vi "Cam Handler.vi"() -> ()   [LabVIEW 2015]
uses:
  <vilib>/userdefined/High Color/IMAQdx.ctl
  <vilib>/vision/driver/NI_Vision_Acquisition_Software.lvlib
  <resource>/objmgr/imaqdx.rc
  <resource>/objmgr/IMAQImage.rc
panel:
  out "Image Size":cluster{"x":i32, "y":i32}
  in  "stop":bool
  out "error out 2":errorcluster
  out "error out":errorcluster
  out "Image Out":T1(plugin-control)
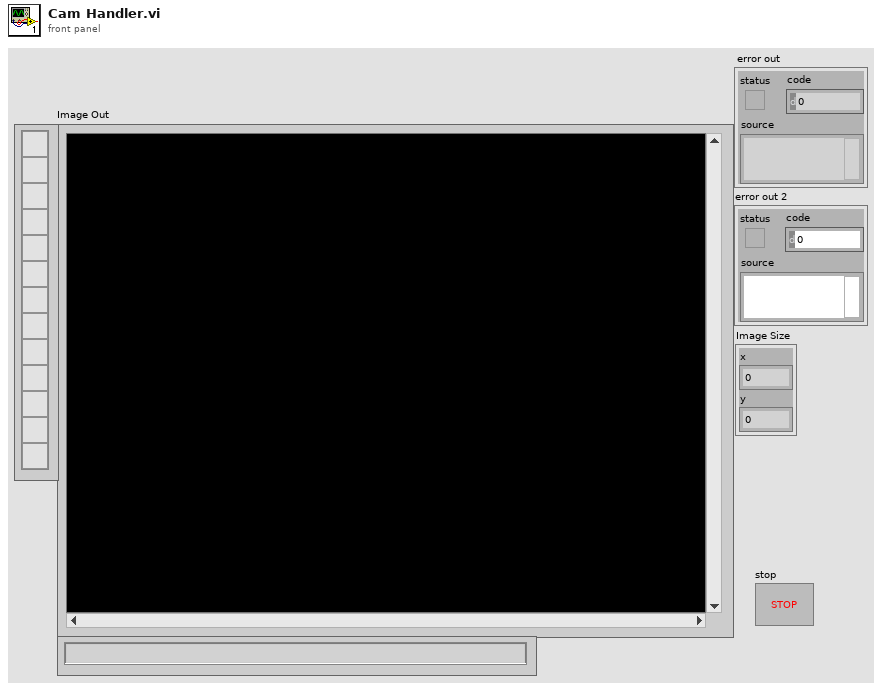
[diagram p1: front panel]
types:
  T1 = typedef "IMAQ Image.ctl" = refnum<image>
  T2 = typedef "IMAQdx.ctl" = refnum<k21>
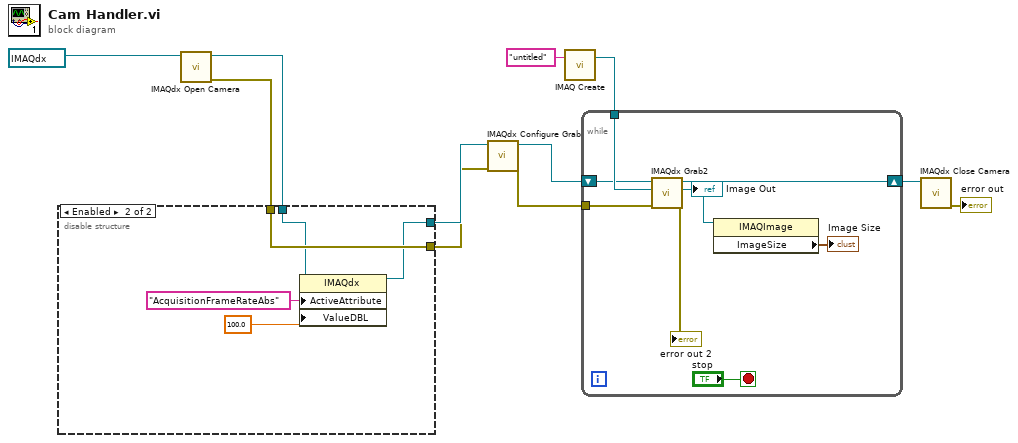
[diagram p0: block diagram]
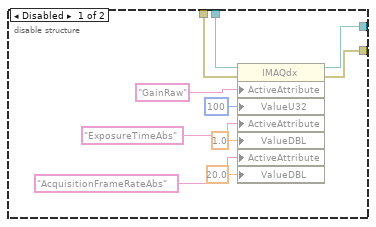
[diagram p2: hidden frame]
diagram:
  n1 = call <vilib>:"IMAQdx Open Camera.vi"("Session In"=T2 "cam1") -> ("error out"=w11:errorcluster, "Session Out"=w10:T2)  [unwired: 9 in]
  n2 = disable-structure shown="Enabled" {
    disable-tunnel: w11 -> [w21 w26]
    disable-tunnel: w10 -> [w20 w25]
    disable-tunnel: [w19 w24] -> w8
    disable-tunnel: [w18 w26] -> w7
    frame Disabled {
      n3 = property class="IMAQdx"(reference=w20, error in=w21, "ActiveAttribute"="GainRaw", "ValueU32"=u32 100, "ActiveAttribute"="ExposureTimeAbs", "ValueDBL"=1.0, "ActiveAttribute"="AcquisitionFrameRateAbs", "ValueDBL"=20.0) -> (reference out=w19:T2, error out=w18:errorcluster)
    }
    frame Enabled {
      n4 = property class="IMAQdx"(reference=w25, "ActiveAttribute"="AcquisitionFrameRateAbs", "ValueDBL"=100.0) -> (reference out=w24:T2)  [unwired: 1 in, 1 out]
    }
  }
  n5 = call <vilib>:"IMAQdx Configure Grab.vi"("error in"=w7, "Session In"=w8) -> ("error out"=w1:errorcluster, "Session Out"=w5:T2)  [unwired: 8 in]
  n6 = call "IMAQ Create"("Image Name"="untitled") -> ("New Image"=w6:T1)  [unwired: 4 in, 1 out]
  n7 = while {
    tunnel: w6 -> [w34]
    shift-right: [w32] -> w4
    shift-left: w5 -> [w33]
    tunnel: w1 -> [w29]
    stop <- "stop" stop-if-true
    n8 = call <vilib>:"IMAQdx Grab2.vi"("error in"=w29, "Image In"=w34, "Session In"=w33) -> ("error out"=→"error out 2":errorcluster, "Image Out"=w28:T1, "Session Out"=w32:T2)  [unwired: 5 in, 1 out]
    "Image Out" <- w28
    n9 = property class="IMAQImage"(reference=w28) -> ("ImageSize"=→"Image Size":cluster{"x":i32, "y":i32})  [unwired: 1 in, 2 out]
  }
  n10 = call <vilib>:"IMAQdx Close Camera.vi"("Session In"=w4) -> ("error out"=→"error out":errorcluster)  [unwired: 10 in]
